vi "test TCX read (installed 71).vi"() -> ()   [LabVIEW 2011] (continued)
</LatitudeDegrees><LongitudeDegrees>-78.914795</LongitudeDegrees></Position><AltitudeMeters>81.849</AltitudeMeters><DistanceMeters>6281.057</DistanceMeters><Cadence>66</Cadence><Extensions><TPX xmlns=\"http://www.garmin.com/xmlschemas/ActivityExtension/v2\"><Watts>174</Watts></TPX></Extensions></Trackpoint><Trackpoint><Time>2008-03-03T13:59:48Z</Time><Position><LatitudeDegrees>35.867644</LatitudeDegrees><LongitudeDegrees>-78.914794</LongitudeDegrees></Position><AltitudeMeters>81.849</AltitudeMeters><DistanceMeters>6288.618</DistanceMeters><Cadence>66</Cadence><Extensions><TPX xmlns=\"http://www.garmin.com/xmlschemas/ActivityExtension/v2\"><Watts>174</Watts></TPX></Extensions></Trackpoint><Trackpoint><Time>2008-03-03T13:59:49Z</Time><Position><LatitudeDegrees>35.867574</LatitudeDegrees><LongitudeDegrees>-78.914794</LongitudeDegrees></Position><AltitudeMeters>82.330</AltitudeMeters><DistanceMeters>6296.373</DistanceMeters><Cadence>65</Cadence><Extensions><TPX xmlns=\"http://www.garmin.com/xmlschemas/ActivityExtension/v2\"><Watts>173</Watts></TPX></Extensions></Trackpoint><Trackpoint><Time>2008-03-03T13:59:50Z</Time><Position><LatitudeDegrees>35.867508</LatitudeDegrees><LongitudeDegrees>-78.914800</LongitudeDegrees></Position><AltitudeMeters>82.330</AltitudeMeters><DistanceMeters>6303.681</DistanceMeters><Cadence>65</Cadence><Extensions><TPX xmlns=\"http://www.garmin.com/xmlschemas/ActivityExtension/v2\"><Watts>179</Watts></TPX></Extensions></Trackpoint><Trackpoint><Time>2008-03-03T13:59:51Z</Time><Position><LatitudeDegrees>35.867435</LatitudeDegrees><LongitudeDegrees>-78.914803</LongitudeDegrees></Position><AltitudeMeters>82.330</AltitudeMeters><DistanceMeters>6311.776</DistanceMeters><Cadence>66</Cadence><Extensions><TPX xmlns=\"http://www.garmin.com/xmlschemas/ActivityExtension/v2\"><Watts>180</Watts></TPX></Extensions></Trackpoint><Trackpoint><Time>2008-03-03T13:59:52Z</Time><Position><LatitudeDegrees>35.867371</LatitudeDegrees><LongitudeDegrees>-78.914809</LongitudeDegrees></Position><AltitudeMeters>82.811</AltitudeMeters><DistanceMeters>6318.962</DistanceMeters><Cadence>65</Cadence><Extensions><TPX xmlns=\"http://www.garmin.com/xmlschemas/ActivityExtension/v2\"><Watts>178</Watts></TPX></Extensions></Trackpoint><Trackpoint><Time>2008-03-03T13:59:53Z</Time><Position><LatitudeDegrees>35.867318</LatitudeDegrees><LongitudeDegrees>-78.914827</LongitudeDegrees></Position><AltitudeMeters>82.330</AltitudeMeters><DistanceMeters>6324.954</DistanceMeters><Cadence>65</Cadence><Extensions><TPX xmlns=\"http://www.garmin.com/xmlschemas/ActivityExtension/v2\"><Watts>191</Watts></TPX></Extensions></Trackpoint><Trackpoint><Time>2008-03-03T13:59:54Z</Time><Position><LatitudeDegrees>35.867262</LatitudeDegrees><LongitudeDegrees>-78.914850</LongitudeDegrees></Position><AltitudeMeters>82.811</AltitudeMeters><DistanceMeters>6331.504</DistanceMeters><Cadence>65</Cadence><Extensions><TPX xmlns=\"http://www.garmin.com/xmlschemas/ActivityExtension/v2\"><Watts>186</Watts></TPX></Extensions></Trackpoint><Trackpoint><Time>2008-03-03T13:59:55Z</Time><Position><LatitudeDegrees>35.867202</LatitudeDegrees><LongitudeDegrees>-78.914873</LongitudeDegrees></Position><AltitudeMeters>82.811</AltitudeMeters><DistanceMeters>6338.441</DistanceMeters><Cadence>64</Cadence><Extensions><TPX xmlns=\"http://www.garmin.com/xmlschemas/ActivityExtension/v2\"><Watts>196</Watts></TPX></Extensions></Trackpoint><Trackpoint><Time>2008-03-03T13:59:57Z</Time><Position><LatitudeDegrees>35.867088</LatitudeDegrees><LongitudeDegrees>-78.914924</LongitudeDegrees></Position><AltitudeMeters>82.811</AltitudeMeters><DistanceMeters>6354.206</DistanceMeters><Cadence>63</Cadence><Extensions><TPX xmlns=\"http://www.garmin.com/xmlschemas/ActivityExtension/v2\"><Watts>82</Watts></TPX></Extensions></Trackpoint><Trackpoint><Time>2008-03-03T13:59:58Z</Time><Position><LatitudeDegrees>35.867029</LatitudeDegrees><LongitudeDegrees>-78.914948</LongitudeDegrees></Position><AltitudeMeters>82.811</AltitudeMeters><DistanceMeters>6358.836</DistanceMeters><Cadence>63</Cadence><Extensions><TPX xmlns=\"http://www.garmin.com/xmlschemas/ActivityExtension/v2\"><Watts>297</Watts></TPX></Extensions></Trackpoint><Trackpoint><Time>2008-03-03T13:59:59Z</Time><Position><LatitudeDegrees>35.866977</LatitudeDegrees><LongitudeDegrees>-78.914975</LongitudeDegrees></Position><AltitudeMeters>82.811</AltitudeMeters><DistanceMeters>6364.992</DistanceMeters><Cadence>65</Cadence><Extensions><TPX xmlns=\"http://www.garmin.com/xmlschemas/ActivityExtension/v2\"><Watts>183</Watts></TPX></Extensions></Trackpoint><Trackpoint><Time>2008-03-03T14:00:00Z</Time><Position><LatitudeDegrees>35.866928</LatitudeDegrees><LongitudeDegrees>-78.915004</LongitudeDegrees></Position><AltitudeMeters>83.291</AltitudeMeters><DistanceMeters>6371.066</DistanceMeters><Cadence>68</Cadence><Extensions><TPX xmlns=\"http://www.garmin.com/xmlschemas/ActivityExtension/v2\"><Watts>185</Watts></TPX></Extensions></Trackpoint><Trackpoint><Time>2008-03-03T14:00:01Z</Time><Position><LatitudeDegrees>35.866873</LatitudeDegrees><LongitudeDegrees>-78.915034</LongitudeDegrees></Position><AltitudeMeters>83.291</AltitudeMeters><DistanceMeters>6377.685</DistanceMeters><Cadence>69</Cadence><Extensions><TPX xmlns=\"http://www.garmin.com/xmlschemas/ActivityExtension/v2\"><Watts>217</Watts></TPX></Extensions></Trackpoint><Trackpoint><Time>2008-03-03T14:00:02Z</Time><Position><LatitudeDegrees>35.866819</LatitudeDegrees><LongitudeDegrees>-78.915064</LongitudeDegrees></Position><AltitudeMeters>83.772</AltitudeMeters><DistanceMeters>6384.382</DistanceMeters><Cadence>70</Cadence><Extensions><TPX xmlns=\"http://www.garmin.com/xmlschemas/ActivityExtension/v2\"><Watts>307</Watts></TPX></Extensions></Trackpoint><Trackpoint><Time>2008-03-03T14:00:03Z</Time><Position><LatitudeDegrees>35.866764</LatitudeDegrees><LongitudeDegrees>-78.915096</LongitudeDegrees></Position><AltitudeMeters>83.772</AltitudeMeters><DistanceMeters>6391.124</DistanceMeters><Cadence>72</Cadence><Extensions><TPX xmlns=\"http://www.garmin.com/xmlschemas/ActivityExtension/v2\"><Watts>372</Watts></TPX></Extensions></Trackpoint><Trackpoint><Time>2008-03-03T14:00:04Z</Time><Position><LatitudeDegrees>35.866708</LatitudeDegrees><LongitudeDegrees>-78.915128</LongitudeDegrees></Position><AltitudeMeters>84.253</AltitudeMeters><DistanceMeters>6397.889</DistanceMeters><Cadence>75</Cadence><Extensions><TPX xmlns=\"http://www.garmin.com/xmlschemas/ActivityExtension/v2\"><Watts>385</Watts></TPX></Extensions></Trackpoint><Trackpoint><Time>2008-03-03T14:00:05Z</Time><Position><LatitudeDegrees>35.866647</LatitudeDegrees><LongitudeDegrees>-78.915159</LongitudeDegrees></Position><AltitudeMeters>84.253</AltitudeMeters><DistanceMeters>6405.212</DistanceMeters><Cadence>75</Cadence><Extensions><TPX xmlns=\"http://www.garmin.com/xmlschemas/ActivityExtension/v2\"><Watts>349</Watts></TPX></Extensions></Trackpoint><Trackpoint><Time>2008-03-03T14:00:06Z</Time><Position><LatitudeDegrees>35.866589</LatitudeDegrees><LongitudeDegrees>-78.915188</LongitudeDegrees></Position><AltitudeMeters>84.733</AltitudeMeters><DistanceMeters>6412.198</DistanceMeters><Cadence>74</Cadence><Extensions><TPX xmlns=\"http://www.garmin.com/xmlschemas/ActivityExtension/v2\"><Watts>306</Watts></TPX></Extensions></Trackpoint><Trackpoint><Time>2008-03-03T14:00:07Z</Time><Position><LatitudeDegrees>35.866529</LatitudeDegrees><LongitudeDegrees>-78.915213</LongitudeDegrees></Position><AltitudeMeters>84.733</AltitudeMeters><DistanceMeters>6419.209</DistanceMeters><Cadence>73</Cadence><Extensions><TPX xmlns=\"http://www.garmin.com/xmlschemas/ActivityExtension/v2\"><Watts>284</Watts></TPX></Extensions></Trackpoint><Trackpoint><Time>2008-03-03T14:00:08Z</Time><Position><LatitudeDegrees>35.866467</LatitudeDegrees><LongitudeDegrees>-78.915237</LongitudeDegrees></Position><AltitudeMeters>84.733</AltitudeMeters><DistanceMeters>6426.446</DistanceMeters><Cadence>73</Cadence><Extensions><TPX xmlns=\"http://www.garmin.com/xmlschemas/ActivityExtension/v2\"><Watts>284</Watts></TPX></Extensions></Trackpoint><Trackpoint><Time>2008-03-03T14:00:09Z</Time><Position><LatitudeDegrees>35.866403</LatitudeDegrees><LongitudeDegrees>-78.915259</LongitudeDegrees></Position><AltitudeMeters>84.733</AltitudeMeters><DistanceMeters>6433.845</DistanceMeters><Cadence>71</Cadence><Extensions><TPX xmlns=\"http://www.garmin.com/xmlschemas/ActivityExtension/v2\"><Watts>278</Watts></TPX></Extensions></Trackpoint><Trackpoint><Time>2008-03-03T14:00:10Z</Time><Position><LatitudeDegrees>35.866343</LatitudeDegrees><LongitudeDegrees>-78.915280</LongitudeDegrees></Position><AltitudeMeters>85.214</AltitudeMeters><DistanceMeters>6440.732</DistanceMeters><Cadence>70</Cadence><Extensions><TPX xmlns=\"http://www.garmin.com/xmlschemas/ActivityExtension/v2\"><Watts>277</Watts></TPX></Extensions></Trackpoint><Trackpoint><Time>2008-03-03T14:00:11Z</Time><Position><LatitudeDegrees>35.866283</LatitudeDegrees><LongitudeDegrees>-78.915301</LongitudeDegrees></Position><AltitudeMeters>85.214</AltitudeMeters><DistanceMeters>6447.618</DistanceMeters><Cadence>70</Cadence><Extensions><TPX xmlns=\"http://www.garmin.com/xmlschemas/ActivityExtension/v2\"><Watts>278</Watts></TPX></Extensions></Trackpoint><Trackpoint><Time>2008-03-03T14:00:12Z</Time><Position><LatitudeDegrees>35.866224</LatitudeDegrees><LongitudeDegrees>-78.915319</LongitudeDegrees></Position><AltitudeMeters>85.695</AltitudeMeters><DistanceMeters>6454.418</DistanceMeters><Cadence>69</Cadence><Extensions><TPX xmlns=\"http://www.garmin.com/xmlschemas/ActivityExtension/v2\"><Watts>278</Watts></TPX></Extensions></Trackpoint><Trackpoint><Time>2008-03-03T14:00:13Z</Time><Position><LatitudeDegrees>35.866163</LatitudeDegrees><LongitudeDegrees>-78.915335</LongitudeDegrees></Position><AltitudeMeters>85.695</AltitudeMeters><DistanceMeters>6461.310</DistanceMeters><Cadence>70</Cadence><Extensions><TPX xmlns=\"http://www.garmin.com/xmlschemas/ActivityExtension/v2\"><Watts>239</Watts></TPX></Extensions></Trackpoint><Trackpoint><Time>2008-03-03T14:00:14Z</Time><Position><LatitudeDegrees>35.866102</LatitudeDegrees><LongitudeDegrees>-78.915349</LongitudeDegrees></Position><AltitudeMeters>85.695</AltitudeMeters><DistanceMeters>6468.183</DistanceMeters><Cadence>71</Cadence><Extensions><TPX xmlns=\"http://www.garmin.com/xmlschemas/ActivityExtension/v2\"><Watts>204</Watts></TPX></Extensions></Trackpoint><Trackpoint><Time>2008-03-03T14:00:15Z</Time><Position><LatitudeDegrees>35.866039</LatitudeDegrees><LongitudeDegrees>-78.915359</LongitudeDegrees></Position><AltitudeMeters>85.695</AltitudeMeters><DistanceMeters>6475.289</DistanceMeters><Cadence>72</Cadence><Extensions><TPX xmlns=\"http://www.garmin.com/xmlschemas/ActivityExtension/v2\"><Watts>186</Watts></TPX></Extensions></Trackpoint><Trackpoint><Time>2008-03-03T14:00:16Z</Time><Position><LatitudeDegrees>35.865974</LatitudeDegrees><LongitudeDegrees>-78.915370</LongitudeDegrees></Position><AltitudeMeters>85.695</AltitudeMeters><DistanceMeters>6482.545</DistanceMeters><Cadence>73</Cadence><Extensions><TPX xmlns=\"http://www.garmin.com/xmlschemas/ActivityExtension/v2\"><Watts>172</Watts></TPX></Extensions></Trackpoint><Trackpoint><Time>2008-03-03T14:00:17Z</Time><Position><LatitudeDegrees>35.865907</LatitudeDegrees><LongitudeDegrees>-78.915378</LongitudeDegrees></Position><AltitudeMeters>85.214</AltitudeMeters><DistanceMeters>6489.986</DistanceMeters><Cadence>75</Cadence><Extensions><TPX xmlns=\"http://www.garmin.com/xmlschemas/ActivityExtension/v2\"><Watts>137</Watts></TPX></Extensions></Trackpoint><Trackpoint><Time>2008-03-03T14:00:18Z</Time><Position><LatitudeDegrees>35.865835</LatitudeDegrees><LongitudeDegrees>-78.915383</LongitudeDegrees></Position><AltitudeMeters>85.214</AltitudeMeters><DistanceMeters>6498.098</DistanceMeters><Cadence>75</Cadence><Extensions><TPX xmlns=\"http://www.garmin.com/xmlschemas/ActivityExtension/v2\"><Watts>137</Watts></TPX></Extensions></Trackpoint><Trackpoint><Time>2008-03-03T14:00:19Z</Time><Position><LatitudeDegrees>35.865761</LatitudeDegrees><LongitudeDegrees>-78.915390</LongitudeDegrees></Position><AltitudeMeters>85.214</AltitudeMeters><DistanceMeters>6506.323</DistanceMeters><Cadence>72</Cadence><Extensions><TPX xmlns=\"http://www.garmin.com/xmlschemas/ActivityExtension/v2\"><Watts>133</Watts></TPX></Extensions></Trackpoint><Trackpoint><Time>2008-03-03T14:00:20Z</Time><Position><LatitudeDegrees>35.865689</LatitudeDegrees><LongitudeDegrees>-78.915399</LongitudeDegrees></Position><AltitudeMeters>85.214</AltitudeMeters><DistanceMeters>6514.329</DistanceMeters><Cadence>75</Cadence><Extensions><TPX xmlns=\"http://www.garmin.com/xmlschemas/ActivityExtension/v2\"><Watts>129</Watts></TPX></Extensions></Trackpoint><Trackpoint><Time>2008-03-03T14:00:21Z</Time><Position><LatitudeDegrees>35.865614</LatitudeDegrees><LongitudeDegrees>-78.915408</LongitudeDegrees></Position><AltitudeMeters>85.214</AltitudeMeters><DistanceMeters>6522.741</DistanceMeters><Cadence>77</Cadence><Extensions><TPX xmlns=\"http://www.garmin.com/xmlschemas/ActivityExtension/v2\"><Watts>129</Watts></TPX></Extensions></Trackpoint><Trackpoint><Time>2008-03-03T14:00:22Z</Time><Position><LatitudeDegrees>35.865534</LatitudeDegrees><LongitudeDegrees>-78.915417</LongitudeDegrees></Position><AltitudeMeters>84.733</AltitudeMeters><DistanceMeters>6531.653</DistanceMeters><Cadence>80</Cadence><Extensions><TPX xmlns=\"http://www.garmin.com/xmlschemas/ActivityExtension/v2\"><Watts>106</Watts></TPX></Extensions></Trackpoint><Trackpoint><Time>2008-03-03T14:00:23Z</Time><Position><LatitudeDegrees>35.865456</LatitudeDegrees><LongitudeDegrees>-78.915429</LongitudeDegrees></Position><AltitudeMeters>84.253</AltitudeMeters><DistanceMeters>6540.289</DistanceMeters><Cadence>80</Cadence><Extensions><TPX xmlns=\"http://www.garmin.com/xmlschemas/ActivityExtension/v2\"><Watts>106</Watts></TPX></Extensions></Trackpoint><Trackpoint><Time>2008-03-03T14:00:24Z</Time><Position><LatitudeDegrees>35.865376</LatitudeDegrees><LongitudeDegrees>-78.915441</LongitudeDegrees></Position><AltitudeMeters>84.253</AltitudeMeters><DistanceMeters>6549.295</DistanceMeters><Cadence>84</Cadence><Extensions><TPX xmlns=\"http://www.garmin.com/xmlschemas/ActivityExtension/v2\"><Watts>98</Watts></TPX></Extensions></Trackpoint><Trackpoint><Time>2008-03-03T14:00:25Z</Time><Position><LatitudeDegrees>35.865294</LatitudeDegrees><LongitudeDegrees>-78.915453</LongitudeDegrees></Position><AltitudeMeters>83.772</AltitudeMeters><DistanceMeters>6558.491</DistanceMeters><Cadence>84</Cadence><Extensions><TPX xmlns=\"http://www.garmin.com/xmlschemas/ActivityExtension/v2\"><Watts>97</Watts></TPX></Extensions></Trackpoint><Trackpoint><Time>2008-03-03T14:00:26Z</Time><Position><LatitudeDegrees>35.865210</LatitudeDegrees><LongitudeDegrees>-78.915464</LongitudeDegrees></Position><AltitudeMeters>83.772</AltitudeMeters><DistanceMeters>6567.843</DistanceMeters><Cadence>81</Cadence><Extensions><TPX xmlns=\"http://www.garmin.com/xmlschemas/ActivityExtension/v2\"><Watts>98</Watts></TPX></Extensions></Trackpoint><Trackpoint><Time>2008-03-03T14:00:27Z</Time><Position><LatitudeDegrees>35.865125</LatitudeDegrees><LongitudeDegrees>-78.915474</LongitudeDegrees></Position><AltitudeMeters>83.291</AltitudeMeters><DistanceMeters>6577.356</DistanceMeters><Cadence>77</Cadence><Extensions><TPX xmlns=\"http://www.garmin.com/xmlschemas/ActivityExtension/v2\"><Watts>93</Watts></TPX></Extensions></Trackpoint><Trackpoint><Time>2008-03-03T14:00:28Z</Time><Position><LatitudeDegrees>35.865038</LatitudeDegrees><LongitudeDegrees>-78.915484</LongitudeDegrees></Position><AltitudeMeters>83.291</AltitudeMeters><DistanceMeters>6587.091</DistanceMeters><Cadence>78</Cadence><Extensions><TPX xmlns=\"http://www.garmin.com/xmlschemas/ActivityExtension/v2\"><Watts>98</Watts></TPX></Extensions></Trackpoint><Trackpoint><Time>2008-03-03T14:00:29Z</Time><Position><LatitudeDegrees>35.864950</LatitudeDegrees><LongitudeDegrees>-78.915492</LongitudeDegrees></Position><AltitudeMeters>83.291</AltitudeMeters><DistanceMeters>6596.888</DistanceMeters><Cadence>79</Cadence><Extensions><TPX xmlns=\"http://www.garmin.com/xmlschemas/ActivityExtension/v2\"><Watts>101</Watts></TPX></Extensions></Trackpoint><Trackpoint><Time>2008-03-03T14:00:30Z</Time><Position><LatitudeDegrees>35.864860</LatitudeDegrees><LongitudeDegrees>-78.915492</LongitudeDegrees></Position><AltitudeMeters>82.811</AltitudeMeters><DistanceMeters>6606.776</DistanceMeters><Cadence>79</Cadence><Extensions><TPX xmlns=\"http://www.garmin.com/xmlschemas/ActivityExtension/v2\"><Watts>100</Watts></TPX></Extensions></Trackpoint><Trackpoint><Time>2008-03-03T14:00:31Z</Time><Position><LatitudeDegrees>35.864773</LatitudeDegrees><LongitudeDegrees>-78.915474</LongitudeDegrees></Position><AltitudeMeters>82.330</AltitudeMeters><DistanceMeters>6616.604</DistanceMeters><Cadence>81</Cadence><Extensions><TPX xmlns=\"http://www.garmin.com/xmlschemas/ActivityExtension/v2\"><Watts>90</Watts></TPX></Extensions></Trackpoint><Trackpoint><Time>2008-03-03T14:00:32Z</Time><Position><LatitudeDegrees>35.864692</LatitudeDegrees><LongitudeDegrees>-78.915428</LongitudeDegrees></Position><AltitudeMeters>81.849</AltitudeMeters><DistanceMeters>6626.400</DistanceMeters><Cadence>81</Cadence><Extensions><TPX xmlns=\"http://www.garmin.com/xmlschemas/ActivityExtension/v2\"><Watts>85</Watts></TPX></Extensions></Trackpoint><Trackpoint><Time>2008-03-03T14:00:33Z</Time><Position><LatitudeDegrees>35.864620</LatitudeDegrees><LongitudeDegrees>-78.915355</LongitudeDegrees></Position><AltitudeMeters>81.369</AltitudeMeters><DistanceMeters>6636.802</DistanceMeters><Cadence>82</Cadence><Extensions><TPX xmlns=\"http://www.garmin.com/xmlschemas/ActivityExtension/v2\"><Watts>85</Watts></TPX></Extensions></Trackpoint><Trackpoint><Time>2008-03-03T14:00:34Z</Time><Position><LatitudeDegrees>35.864573</LatitudeDegrees><LongitudeDegrees>-78.915260</LongitudeDegrees></Position><AltitudeMeters>80.888</AltitudeMeters><DistanceMeters>6646.822</DistanceMeters><Cadence>82</Cadence><Extensions><TPX xmlns=\"http://www.garmin.com/xmlschemas/ActivityExtension/v2\"><Watts>88</Watts></TPX></Extensions></Trackpoint><Trackpoint><Time>2008-03-03T14:00:35Z</Time><Position><LatitudeDegrees>35.864537</LatitudeDegrees><LongitudeDegrees>-78.915158</LongitudeDegrees></Position><AltitudeMeters>80.888</AltitudeMeters><DistanceMeters>6656.818</DistanceMeters><Cadence>82</Cadence><Extensions><TPX xmlns=\"http://www.garmin.com/xmlschemas/ActivityExtension/v2\"><Watts>89</Watts></TPX></Extensions></Trackpoint><Trackpoint><Time>2008-03-03T14:00:36Z</Time><Position><LatitudeDegrees>35.864505</LatitudeDegrees><LongitudeDegrees>-78.915054</LongitudeDegrees></Position><AltitudeMeters>80.888</AltitudeMeters><DistanceMeters>6666.811</DistanceMeters><Cadence>79</Cadence><Extensions><TPX xmlns=\"http://www.garmin.com/xmlschemas/ActivityExtension/v2\"><Watts>91</Watts></TPX></Extensions></Trackpoint><Trackpoint><Time>2008-03-03T14:00:37Z</Time><Position><LatitudeDegrees>35.864475</LatitudeDegrees><LongitudeDegrees>-78.914951</LongitudeDegrees></Position><AltitudeMeters>80.888</AltitudeMeters><DistanceMeters>6676.699</DistanceMeters><Cadence>79</Cadence><Extensions><TPX xmlns=\"http://www.garmin.com/xmlschemas/ActivityExtension/v2\"><Watts>91</Watts></TPX></Extensions></Trackpoint><Trackpoint><Time>2008-03-03T14:00:38Z</Time><Position><LatitudeDegrees>35.864448</LatitudeDegrees><LongitudeDegrees>-78.914848</LongitudeDegrees></Position><AltitudeMeters>80.888</AltitudeMeters><DistanceMeters>6686.446</DistanceMeters><Cadence>76</Cadence><Extensions><TPX xmlns=\"http://www.garmin.com/xmlschemas/ActivityExtension/v2\"><Watts>91</Watts></TPX></Extensions></Trackpoint><Trackpoint><Time>2008-03-03T14:00:39Z</Time><Position><LatitudeDegrees>35.864423</LatitudeDegrees><LongitudeDegrees>-78.914748</LongitudeDegrees></Position><AltitudeMeters>80.888</AltitudeMeters><DistanceMeters>6695.848</DistanceMeters><Cadence>75</Cadence><Extensions><TPX xmlns=\"http://www.garmin.com/xmlschemas/ActivityExtension/v2\"><Watts>102</Watts></TPX></Extensions></Trackpoint><Trackpoint><Time>2008-03-03T14:00:40Z</Time><Position><LatitudeDegrees>35.864400</LatitudeDegrees><LongitudeDegrees>-78.914650</LongitudeDegrees></Position><AltitudeMeters>80.888</AltitudeMeters><DistanceMeters>6704.998</DistanceMeters><Cadence>73</Cadence><Extensions><TPX xmlns=\"http://www.garmin.com/xmlschemas/ActivityExtension/v2\"><Watts>117</Watts></TPX></Extensions></Trackpoint><Trackpoint><Time>2008-03-03T14:00:41Z</Time><Position><LatitudeDegrees>35.864383</LatitudeDegrees><LongitudeDegrees>-78.914555</LongitudeDegrees></Position><AltitudeMeters>80.888</AltitudeMeters><DistanceMeters>6713.747</DistanceMeters><Cadence>68</Cadence><Extensions><TPX xmlns=\"http://www.garmin.com/xmlschemas/ActivityExtension/v2\"><Watts>151</Watts></TPX></Extensions></Trackpoint><Trackpoint><Time>2008-03-03T14:00:42Z</Time><Position><LatitudeDegrees>35.864372</LatitudeDegrees><LongitudeDegrees>-78.914466</LongitudeDegrees></Position><AltitudeMeters>81.369</AltitudeMeters><DistanceMeters>6721.860</DistanceMeters><Cadence>70</Cadence><Extensions><TPX xmlns=\"http://www.garmin.com/xmlschemas/ActivityExtension/v2\"><Watts>150</Watts></TPX></Extensions></Trackpoint><Trackpoint><Time>2008-03-03T14:00:43Z</Time><Position><LatitudeDegrees>35.864359</LatitudeDegrees><LongitudeDegrees>-78.914380</LongitudeDegrees></Position><AltitudeMeters>81.369</AltitudeMeters><DistanceMeters>6729.762</DistanceMeters><Cadence>80</Cadence><Extensions><TPX xmlns=\"http://www.garmin.com/xmlschemas/ActivityExtension/v2\"><Watts>145</Watts></TPX></Extensions></Trackpoint><Trackpoint><Time>2008-03-03T14:00:44Z</Time><Position><LatitudeDegrees>35.864347</LatitudeDegrees><LongitudeDegrees>-78.914297</LongitudeDegrees></Position><AltitudeMeters>81.849</AltitudeMeters><DistanceMeters>6737.294</DistanceMeters><Cadence>77</Cadence><Extensions><TPX xmlns=\"http://www.garmin.com/xmlschemas/ActivityExtension/v2\"><Watts>171</Watts></TPX></Extensions></Trackpoint><Trackpoint><Time>2008-03-03T14:00:45Z</Time><Position><LatitudeDegrees>35.864343</LatitudeDegrees><LongitudeDegrees>-78.914218</LongitudeDegrees></Position><AltitudeMeters>81.849</AltitudeMeters><DistanceMeters>6744.497</DistanceMeters><Cadence>76</Cadence><Extensions><TPX xmlns=\"http://www.garmin.com/xmlschemas/ActivityExtension/v2\"><Watts>213</Watts></TPX></Extensions></Trackpoint><Trackpoint><Time>2008-03-03T14:00:46Z</Time><Position><LatitudeDegrees>35.864331</LatitudeDegrees><LongitudeDegrees>-78.914140</LongitudeDegrees></Position><AltitudeMeters>82.330</AltitudeMeters><DistanceMeters>6751.655</DistanceMeters><Cadence>72</Cadence><Extensions><TPX xmlns=\"http://www.garmin.com/xmlschemas/ActivityExtension/v2\"><Watts>272</Watts></TPX></Extensions></Trackpoint><Trackpoint><Time>2008-03-03T14:00:47Z</Time><Position><LatitudeDegrees>35.864314</LatitudeDegrees><LongitudeDegrees>-78.914064</LongitudeDegrees></Position><AltitudeMeters>82.811</AltitudeMeters><DistanceMeters>6758.766</DistanceMeters><Cadence>72</Cadence><Extensions><TPX xmlns=\"http://www.garmin.com/xmlschemas/ActivityExtension/v2\"><Watts>272</Watts></TPX></Extensions></Trackpoint><Trackpoint><Time>2008-03-03T14:00:48Z</Time><Position><LatitudeDegrees>35.864283</LatitudeDegrees><LongitudeDegrees>-78.913987</LongitudeDegrees></Position><AltitudeMeters>83.291</AltitudeMeters><DistanceMeters>6766.340</DistanceMeters><Cadence>71</Cadence><Extensions><TPX xmlns=\"http://www.garmin.com/xmlschemas/ActivityExtension/v2\"><Watts>303</Watts></TPX></Extensions></Trackpoint><Trackpoint><Time>2008-03-03T14:00:49Z</Time><Position><LatitudeDegrees>35.864255</LatitudeDegrees><LongitudeDegrees>-78.913913</LongitudeDegrees></Position><AltitudeMeters>83.291</AltitudeMeters><DistanceMeters>6773.708</DistanceMeters><Cadence>70</Cadence><Extensions><TPX xmlns=\"http://www.garmin.com/xmlschemas/ActivityExtension/v2\"><Watts>304</Watts></TPX></Extensions></Trackpoint><Trackpoint><Time>2008-03-03T14:00:50Z</Time><Position><LatitudeDegrees>35.864235</LatitudeDegrees><LongitudeDegrees>-78.913840</LongitudeDegrees></Position><AltitudeMeters>83.291</AltitudeMeters><DistanceMeters>6780.600</DistanceMeters><Cadence>69</Cadence><Extensions><TPX xmlns=\"http://www.garmin.com/xmlschemas/ActivityExtension/v2\"><Watts>293</Watts></TPX></Extensions></Trackpoint><Trackpoint><Time>2008-03-03T14:00:51Z</Time><Position><LatitudeDegrees>35.864225</LatitudeDegrees><LongitudeDegrees>-78.913771</LongitudeDegrees></Position><AltitudeMeters>83.772</AltitudeMeters><DistanceMeters>6786.828</DistanceMeters><Cadence>67</Cadence><Extensions><TPX xmlns=\"http://www.garmin.com/xmlschemas/ActivityExtension/v2\"><Watts>308</Watts></TPX></Extensions></Trackpoint><Trackpoint><Time>2008-03-03T14:00:52Z</Time><Position><LatitudeDegrees>35.864214</LatitudeDegrees><LongitudeDegrees>-78.913703</LongitudeDegrees></Position><AltitudeMeters>84.253</AltitudeMeters><DistanceMeters>6793.119</DistanceMeters><Cadence>68</Cadence><Extensions><TPX xmlns=\"http://www.garmin.com/xmlschemas/ActivityExtension/v2\"><Watts>370</Watts></TPX></Extensions></Trackpoint><Trackpoint><Time>2008-03-03T14:00:53Z</Time><Position><LatitudeDegrees>35.864201</LatitudeDegrees><LongitudeDegrees>-78.913635</LongitudeDegrees></Position><AltitudeMeters>84.253</AltitudeMeters><DistanceMeters>6799.419</DistanceMeters><Cadence>69</Cadence><Extensions><TPX xmlns=\"http://www.garmin.com/xmlschemas/ActivityExtension/v2\"><Watts>425</Watts></TPX></Extensions></Trackpoint><Trackpoint><Time>2008-03-03T14:00:54Z</Time><Position><LatitudeDegrees>35.864198</LatitudeDegrees><LongitudeDegrees>-78.913567</LongitudeDegrees></Position><AltitudeMeters>84.733</AltitudeMeters><DistanceMeters>6805.544</DistanceMeters><Cadence>68</Cadence><Extensions><TPX xmlns=\"http://www.garmin.com/xmlschemas/ActivityExtension/v2\"><Watts>440</Watts></TPX></Extensions></Trackpoint><Trackpoint><Time>2008-03-03T14:00:55Z</Time><Position><LatitudeDegrees>35.864198</LatitudeDegrees><LongitudeDegrees>-78.913497</LongitudeDegrees></Position><AltitudeMeters>84.733</AltitudeMeters><DistanceMeters>6811.758</DistanceMeters><Cadence>68</Cadence><Extensions><TPX xmlns=\"http://www.garmin.com/xmlschemas/ActivityExtension/v2\"><Watts>438</Watts></TPX></Extensions></Trackpoint><Trackpoint><Time>2008-03-03T14:00:56Z</Time><Position><LatitudeDegrees>35.864194</LatitudeDegrees><LongitudeDegrees>-78.913427</LongitudeDegrees></Position><AltitudeMeters>85.695</AltitudeMeters><DistanceMeters>6818.088</DistanceMeters><Cadence>69</Cadence><Extensions><TPX xmlns=\"http://www.garmin.com/xmlschemas/ActivityExtension/v2\"><Watts>459</Watts></TPX></Extensions></Trackpoint><Trackpoint><Time>2008-03-03T14:00:57Z</Time><Position><LatitudeDegrees>35.864184</LatitudeDegrees><LongitudeDegrees>-78.913356</LongitudeDegrees></Position><AltitudeMeters>86.175</AltitudeMeters><DistanceMeters>6824.570</DistanceMeters><Cadence>70</Cadence><Extensions><TPX xmlns=\"http://www.garmin.com/xmlschemas/ActivityExtension/v2\"><Watts>479</Watts></TPX></Extensions></Trackpoint><Trackpoint><Time>2008-03-03T14:00:58Z</Time><Position><LatitudeDegrees>35.864166</LatitudeDegrees><LongitudeDegrees>-78.913280</LongitudeDegrees></Position><AltitudeMeters>86.175</AltitudeMeters><DistanceMeters>6831.775</DistanceMeters><Cadence>73</Cadence><Extensions><TPX xmlns=\"http://www.garmin.com/xmlschemas/ActivityExtension/v2\"><Watts>598</Watts></TPX></Extensions></Trackpoint><Trackpoint><Time>2008-03-03T14:00:59Z</Time><Position><LatitudeDegrees>35.864150</LatitudeDegrees><LongitudeDegrees>-78.913201</LongitudeDegrees></Position><AltitudeMeters>86.656</AltitudeMeters><DistanceMeters>6839.045</DistanceMeters><Cadence>75</Cadence><Extensions><TPX xmlns=\"http://www.garmin.com/xmlschemas/ActivityExtension/v2\"><Watts>653</Watts></TPX></Extensions></Trackpoint><Trackpoint><Time>2008-03-03T14:01:00Z</Time><Position><LatitudeDegrees>35.864134</LatitudeDegrees><LongitudeDegrees>-78.913121</LongitudeDegrees></Position><AltitudeMeters>87.617</AltitudeMeters><DistanceMeters>6846.459</DistanceMeters><Cadence>76</Cadence><Extensions><TPX xmlns=\"http://www.garmin.com/xmlschemas/ActivityExtension/v2\"><Watts>647</Watts></TPX></Extensions></Trackpoint><Trackpoint><Time>2008-03-03T14:01:01Z</Time><Position><LatitudeDegrees>35.864122</LatitudeDegrees><LongitudeDegrees>-78.913040</LongitudeDegrees></Position><AltitudeMeters>87.137</AltitudeMeters><DistanceMeters>6853.909</DistanceMeters><Cadence>78</Cadence><Extensions><TPX xmlns=\"http://www.garmin.com/xmlschemas/ActivityExtension/v2\"><Watts>700</Watts></TPX></Extensions></Trackpoint><Trackpoint><Time>2008-03-03T14:01:02Z</Time><Position><LatitudeDegrees>35.864111</LatitudeDegrees><LongitudeDegrees>-78.912960</LongitudeDegrees></Position><AltitudeMeters>88.098</AltitudeMeters><DistanceMeters>6861.279</DistanceMeters><Cadence>78</Cadence><Extensions><TPX xmlns=\"http://www.garmin.com/xmlschemas/ActivityExtension/v2\"><Watts>702</Watts></TPX></Extensions></Trackpoint><Trackpoint><Time>2008-03-03T14:01:03Z</Time><Position><LatitudeDegrees>35.864093</LatitudeDegrees><LongitudeDegrees>-78.912875</LongitudeDegrees></Position><AltitudeMeters>88.579</AltitudeMeters><DistanceMeters>6869.185</DistanceMeters><Cadence>80</Cadence><Extensions><TPX xmlns=\"http://www.garmin.com/xmlschemas/ActivityExtension/v2\"><Watts>737</Watts></TPX></Extensions></Trackpoint><Trackpoint><Time>2008-03-03T14:01:04Z</Time><Position><LatitudeDegrees>35.864077</LatitudeDegrees><LongitudeDegrees>-78.912789</LongitudeDegrees></Position><AltitudeMeters>89.540</AltitudeMeters><DistanceMeters>6877.123</DistanceMeters><Cadence>82</Cadence><Extensions><TPX xmlns=\"http://www.garmin.com/xmlschemas/ActivityExtension/v2\"><Watts>748</Watts></TPX></Extensions></Trackpoint><Trackpoint><Time>2008-03-03T14:01:05Z</Time><Position><LatitudeDegrees>35.864060</LatitudeDegrees><LongitudeDegrees>-78.912705</LongitudeDegrees></Position><AltitudeMeters>90.021</AltitudeMeters><DistanceMeters>6884.957</DistanceMeters><Cadence>81</Cadence><Extensions><TPX xmlns=\"http://www.garmin.com/xmlschemas/ActivityExtension/v2\"><Watts>703</Watts></TPX></Extensions></Trackpoint><Trackpoint><Time>2008-03-03T14:01:06Z</Time><Position><LatitudeDegrees>35.864049</LatitudeDegrees><LongitudeDegrees>-78.912624</LongitudeDegrees></Position><AltitudeMeters>90.021</AltitudeMeters><DistanceMeters>6892.311</DistanceMeters><Cadence>81</Cadence><Extensions><TPX xmlns=\"http://www.garmin.com/xmlschemas/ActivityExtension/v2\"><Watts>649</Watts></TPX></Extensions></Trackpoint><Trackpoint><Time>2008-03-03T14:01:07Z</Time><Position><LatitudeDegrees>35.864041</LatitudeDegrees><LongitudeDegrees>-78.912548</LongitudeDegrees></Position><AltitudeMeters>90.982</AltitudeMeters><DistanceMeters>6899.189</DistanceMeters><Cadence>81</Cadence><Extensions><TPX xmlns=\"http://www.garmin.com/xmlschemas/ActivityExtension/v2\"><Watts>642</Watts></TPX></Extensions></Trackpoint><Trackpoint><Time>2008-03-03T14:01:08Z</Time><Position><LatitudeDegrees>35.864020</LatitudeDegrees><LongitudeDegrees>-78.912465</LongitudeDegrees></Position><AltitudeMeters>91.463</AltitudeMeters><DistanceMeters>6907.065</DistanceMeters><Cadence>79</Cadence><Extensions><TPX xmlns=\"http://www.garmin.com/xmlschemas/ActivityExtension/v2\"><Watts>615</Watts></TPX></Extensions></Trackpoint><Trackpoint><Time>2008-03-03T14:01:09Z</Time><Position><LatitudeDegrees>35.864002</LatitudeDegrees><LongitudeDegrees>-78.912381</LongitudeDegrees></Position><AltitudeMeters>92.424</AltitudeMeters><DistanceMeters>6914.858</DistanceMeters><Cadence>79</Cadence><Extensions><TPX xmlns=\"http://www.garmin.com/xmlschemas/ActivityExtension/v2\"><Watts>585</Watts></TPX></Extensions></Trackpoint><Trackpoint><Time>2008-03-03T14:01:10Z</Time><Position><LatitudeDegrees>35.863978</LatitudeDegrees><LongitudeDegrees>-78.912296</LongitudeDegrees></Position><AltitudeMeters>92.905</AltitudeMeters><DistanceMeters>6922.911</DistanceMeters><Cadence>77</Cadence><Extensions><TPX xmlns=\"http://www.garmin.com/xmlschemas/ActivityExtension/v2\"><Watts>553</Watts></TPX></Extensions></Trackpoint><Trackpoint><Time>2008-03-03T14:01:11Z</Time><Position><LatitudeDegrees>35.863964</LatitudeDegrees><LongitudeDegrees>-78.912216</LongitudeDegrees></Position><AltitudeMeters>92.905</AltitudeMeters><DistanceMeters>6930.312</DistanceMeters><Cadence>72</Cadence><Extensions><TPX xmlns=\"http://www.garmin.com/xmlschemas/ActivityExtension/v2\"><Watts>410</Watts></TPX></Extensions></Trackpoint><Trackpoint><Time>2008-03-03T14:01:12Z</Time><Position><LatitudeDegrees>35.863948</LatitudeDegrees><LongitudeDegrees>-78.912141</LongitudeDegrees></Position><AltitudeMeters>93.385</AltitudeMeters><DistanceMeters>6937.269</DistanceMeters><Cadence>72</Cadence><Extensions><TPX xmlns=\"http://www.garmin.com/xmlschemas/ActivityExtension/v2\"><Watts>409</Watts></TPX></Extensions></Trackpoint><Trackpoint><Time>2008-03-03T14:01:13Z</Time><Position><LatitudeDegrees>35.863937</LatitudeDegrees><LongitudeDegrees>-78.912070</LongitudeDegrees></Position><AltitudeMeters>93.385</AltitudeMeters><DistanceMeters>6943.808</DistanceMeters><Cadence>68</Cadence><Extensions><TPX xmlns=\"http://www.garmin.com/xmlschemas/ActivityExtension/v2\"><Watts>307</Watts></TPX></Extensions></Trackpoint><Trackpoint><Time>2008-03-03T14:01:14Z</Time><Position><LatitudeDegrees>35.863933</LatitudeDegrees><LongitudeDegrees>-78.912000</LongitudeDegrees></Position><AltitudeMeters>93.866</AltitudeMeters><DistanceMeters>6950.118</DistanceMeters><Cadence>67</Cadence><Extensions><TPX xmlns=\"http://www.garmin.com/xmlschemas/ActivityExtension/v2\"><Watts>298</Watts></TPX></Extensions></Trackpoint><Trackpoint><Time>2008-03-03T14:01:15Z</Time><Position><LatitudeDegrees>35.863925</LatitudeDegrees><LongitudeDegrees>-78.911930</LongitudeDegrees></Position><AltitudeMeters>93.866</AltitudeMeters><DistanceMeters>6956.486</DistanceMeters><Cadence>66</Cadence><Extensions><TPX xmlns=\"http://www.garmin.com/xmlschemas/ActivityExtension/v2\"><Watts>299</Watts></TPX></Extensions></Trackpoint><Trackpoint><Time>2008-03-03T14:01:16Z</Time><Position><LatitudeDegrees>35.863919</LatitudeDegrees><LongitudeDegrees>-78.911861</LongitudeDegrees></Position><AltitudeMeters>94.347</AltitudeMeters><DistanceMeters>6962.743</DistanceMeters><Cadence>66</Cadence><Extensions><TPX xmlns=\"http://www.garmin.com/xmlschemas/ActivityExtension/v2\"><Watts>282</Watts></TPX></Extensions></Trackpoint><Trackpoint><Time>2008-03-03T14:01:17Z</Time><Position><LatitudeDegrees>35.863914</LatitudeDegrees><LongitudeDegrees>-78.911792</LongitudeDegrees></Position><AltitudeMeters>93.866</AltitudeMeters><DistanceMeters>6969.023</DistanceMeters><Cadence>66</Cadence><Extensions><TPX xmlns=\"http://www.garmin.com/xmlschemas/ActivityExtension/v2\"><Watts>270</Watts></TPX></Extensions></Trackpoint><Trackpoint><Time>2008-03-03T14:01:18Z</Time><Position><LatitudeDegrees>35.863906</LatitudeDegrees><LongitudeDegrees>-78.911721</LongitudeDegrees></Position><AltitudeMeters>93.866</AltitudeMeters><DistanceMeters>6975.491</DistanceMeters><Cadence>67</Cadence><Extensions><TPX xmlns=\"http://www.garmin.com/xmlschemas/ActivityExtension/v2\"><Watts>255</Watts></TPX></Extensions></Trackpoint><Trackpoint><Time>2008-03-03T14:01:19Z</Time><Position><LatitudeDegrees>35.863896</LatitudeDegrees><LongitudeDegrees>-78.911649</LongitudeDegrees></Position><AltitudeMeters>94.347</AltitudeMeters><DistanceMeters>6982.065</DistanceMeters><Cadence>68</Cadence><Extensions><TPX xmlns=\"http://www.garmin.com/xmlschemas/ActivityExtension/v2\"><Watts>227</Watts></TPX></Extensions></Trackpoint><Trackpoint><Time>2008-03-03T14:01:20Z</Time><Position><LatitudeDegrees>35.863886</LatitudeDegrees><LongitudeDegrees>-78.911576</LongitudeDegrees></Position><AltitudeMeters>94.347</AltitudeMeters><DistanceMeters>6988.714</DistanceMeters><Cadence>68</Cadence><Extensions><TPX xmlns=\"http://www.garmin.com/xmlschemas/ActivityExtension/v2\"><Watts>192</Watts></TPX></Extensions></Trackpoint><Trackpoint><Time>2008-03-03T14:01:21Z</Time><Position><LatitudeDegrees>35.863877</LatitudeDegrees><LongitudeDegrees>-78.911503</LongitudeDegrees></Position><AltitudeMeters>94.347</AltitudeMeters><DistanceMeters>6995.386</DistanceMeters><Cadence>70</Cadence><Extensions><TPX xmlns=\"http://www.garmin.com/xmlschemas/ActivityExtension/v2\"><Watts>171</Watts></TPX></Extensions></Trackpoint><Trackpoint><Time>2008-03-03T14:01:22Z</Time><Position><LatitudeDegrees>35.863862</LatitudeDegrees><LongitudeDegrees>-78.911429</LongitudeDegrees></Position><AltitudeMeters>93.866</AltitudeMeters><DistanceMeters>7002.282</DistanceMeters><Cadence>70</Cadence><Extensions><TPX xmlns=\"http://www.garmin.com/xmlschemas/ActivityExtension/v2\"><Watts>169</Watts></TPX></Extensions></Trackpoint><Trackpoint><Time>2008-03-03T14:01:23Z</Time><Position><LatitudeDegrees>35.863847</LatitudeDegrees><LongitudeDegrees>-78.911353</LongitudeDegrees></Position><AltitudeMeters>94.347</AltitudeMeters><DistanceMeters>7009.325</DistanceMeters><Cadence>71</Cadence><Extensions><TPX xmlns=\"http://www.garmin.com/xmlschemas/ActivityExtension/v2\"><Watts>160</Watts></TPX></Extensions></Trackpoint><Trackpoint><Time>2008-03-03T14:01:24Z</Time><Position><LatitudeDegrees>35.863833</LatitudeDegrees><LongitudeDegrees>-78.911275</LongitudeDegrees></Position><AltitudeMeters>93.866</AltitudeMeters><DistanceMeters>7016.554</DistanceMeters><Cadence>73</Cadence><Extensions><TPX xmlns=\"http://www.garmin.com/xmlschemas/ActivityExtension/v2\"><Watts>159</Watts></TPX></Extensions></Trackpoint><Trackpoint><Time>2008-03-03T14:01:25Z</Time><Position><LatitudeDegrees>35.863820</LatitudeDegrees><LongitudeDegrees>-78.911196</LongitudeDegrees></Position><AltitudeMeters>94.347</AltitudeMeters><DistanceMeters>7023.834</DistanceMeters><Cadence>75</Cadence><Extensions><TPX xmlns=\"http://www.garmin.com/xmlschemas/ActivityExtension/v2\"><Watts>150</Watts></TPX></Extensions></Trackpoint><Trackpoint><Time>2008-03-03T14:01:26Z</Time><Position><LatitudeDegrees>35.863806</LatitudeDegrees><LongitudeDegrees>-78.911116</LongitudeDegrees></Position><AltitudeMeters>93.866</AltitudeMeters><DistanceMeters>7031.242</DistanceMeters><Cadence>68</Cadence><Extensions><TPX xmlns=\"http://www.garmin.com/xmlschemas/ActivityExtension/v2\"><Watts>136</Watts></TPX></Extensions></Trackpoint><Trackpoint><Time>2008-03-03T14:01:27Z</Time><Position><LatitudeDegrees>35.863794</LatitudeDegrees><LongitudeDegrees>-78.911035</LongitudeDegrees></Position><AltitudeMeters>93.866</AltitudeMeters><DistanceMeters>7038.731</DistanceMeters><Cadence>70</Cadence><Extensions><TPX xmlns=\"http://www.garmin.com/xmlschemas/ActivityExtension/v2\"><Watts>136</Watts></TPX></Extensions></Trackpoint><Trackpoint><Time>2008-03-03T14:01:28Z</Time><Position><LatitudeDegrees>35.863781</LatitudeDegrees><LongitudeDegrees>-78.910951</LongitudeDegrees></Position><AltitudeMeters>93.866</AltitudeMeters><DistanceMeters>7046.477</DistanceMeters><Cadence>71</Cadence><Extensions><TPX xmlns=\"http://www.garmin.com/xmlschemas/ActivityExtension/v2\"><Watts>133</Watts></TPX></Extensions></Trackpoint><Trackpoint><Time>2008-03-03T14:01:29Z</Time><Position><LatitudeDegrees>35.863764</LatitudeDegrees><LongitudeDegrees>-78.910865</LongitudeDegrees></Position><AltitudeMeters>93.866</AltitudeMeters><DistanceMeters>7054.443</DistanceMeters><Cadence>72</Cadence><Extensions><TPX xmlns=\"http://www.garmin.com/xmlschemas/ActivityExtension/v2\"><Watts>134</Watts></TPX></Extensions></Trackpoint><Trackpoint><Time>2008-03-03T14:01:30Z</Time><Position><LatitudeDegrees>35.863743</LatitudeDegrees><LongitudeDegrees>-78.910777</LongitudeDegrees></Position><AltitudeMeters>93.866</AltitudeMeters><DistanceMeters>7062.775</DistanceMeters><Cadence>75</Cadence><Extensions><TPX xmlns=\"http://www.garmin.com/xmlschemas/ActivityExtension/v2\"><Watts>122</Watts></TPX></Extensions></Trackpoint><Trackpoint><Time>2008-03-03
